vi "helper-log-visa.vi"(11 "VISA REPORT":T2) -> (0 "error out":errorcluster, 3 "array type (2D Dbl)":string[][](array[string]))   [LabVIEW 2024]
uses:
  controls/enum.io.type.ctl
  controls/enum.report-filter.ctl
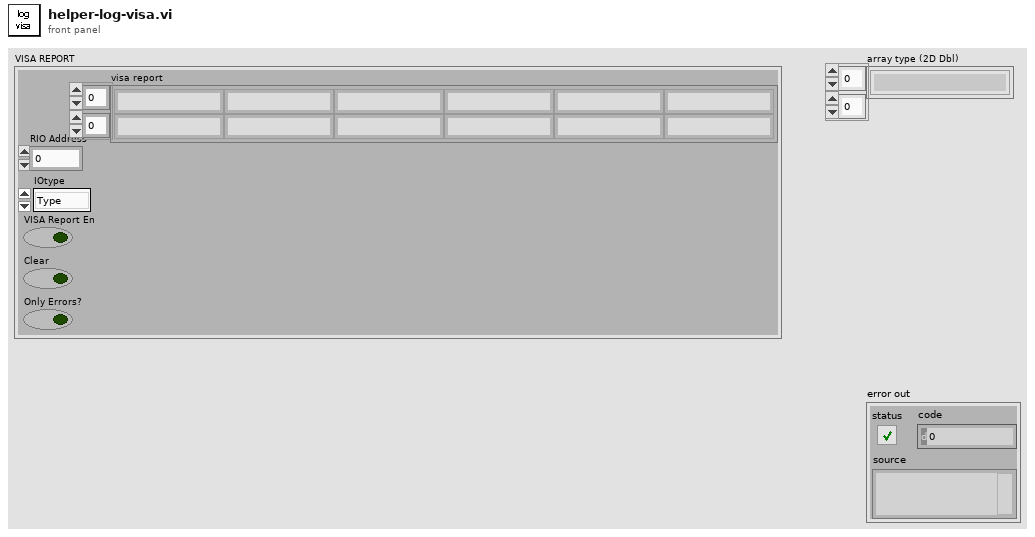
[diagram p1: front panel]
types:
  T1 = typedef "enum.io.type.ctl" = enum16{"Type", "DI", "DO", "AI", "AO", "VL", "BUF"}
  T2 = cluster{"visa report":string[][], "RIO Address":i32, "IOtype":T1, "VISA Report En":bool, "Clear":bool, "Only Errors?":bool}
  T3 = typedef "enum.report-filter.ctl" = enum16{"Read ALL", "Read Errors", "Collect", "ClearAll"}
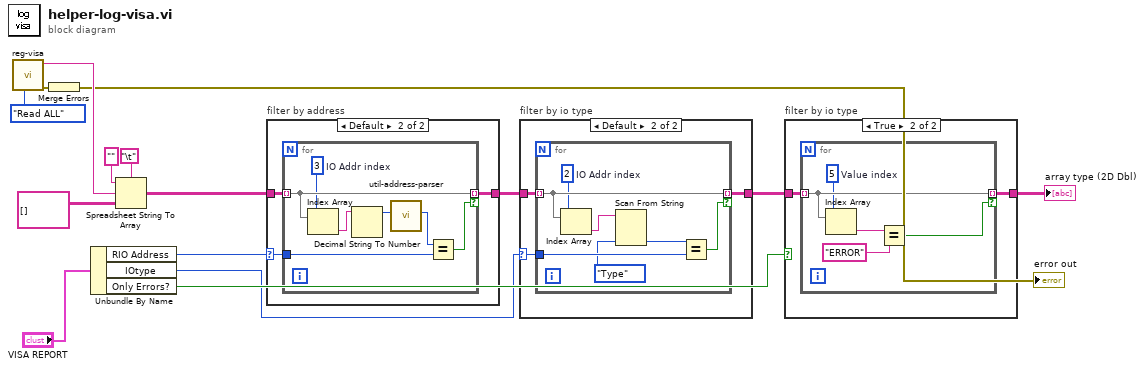
[diagram p0: block diagram]
diagram:
  n1 = call "reg-visa.vi"("Operation(Read)"=enum.report-filter."Read ALL") -> ("error out"=w3:errorcluster, "Collected Reports"=w6:string)  [unwired: 9 in]
  n2 = Merge Errors(w3) -> (→"error out":errorcluster)
  n3 = Unbundle By Name("VISA REPORT") -> ("RIO Address"=w9:i32, "IOtype"=w10:T1, "Only Errors?"=w13:bool)
  n4 = Spreadsheet String To Array(delimiter (Tab)="\t", format string="", spreadsheet string=w6, array type (2D Dbl)=string[][] []) -> (array=w5:string[][])
  n5 = case "filter by address" shown="Default" w9 {
    selector: w9 -> [_ w18]
    tunnel: w5 -> [w16 w19]
    tunnel: [w16 w17] -> w11
    frame ..0 {
    }
    frame Default {
      n6 = for {
        tunnel: w19 -> [w22] mode=indexing
        tunnel: w18 -> [w23]
        tunnel: [w22] -> w17 mode=indexing if=w21
        w20 = 3  # IO Addr index
        n7 = Index Array(array=w22, index=w20) -> (element=w26:string)
        n8 = Decimal String To Number(string=w26) -> (number=w25:i32)  [unwired: 2 in, 1 out]
        n9 = call "util-address-parser.vi"("ADDR 2"=w25) -> ("Address"=w24:u8)  [unwired: 9 in, 1 out]
        n10 = Equal?(x=w24, y=w23) -> (x = y?=w21:bool)
      }
    }
  }
  n11 = case "filter by io type" shown="Default" w10 {
    selector: w10 -> [_ w29]
    tunnel: w11 -> [w27 w30]
    tunnel: [w27 w28] -> w14
    frame "Type" {
    }
    frame Default {
      n12 = for {
        tunnel: w30 -> [w37] mode=indexing
        tunnel: w29 -> [w33]
        tunnel: [w37] -> w28 mode=indexing if=w36
        w35 = 2  # IO Addr index
        n13 = Index Array(array=w37, index=w35) -> (element=w34:string)
        n14 = Scan From String(input string=w34, default 1=enum.io.type."Type" ("IOtype")) -> (output 1=w32:T1)  [unwired: 3 in, 3 out]
        n15 = Equal?(x=w32, y=w33) -> (x = y?=w36:bool)
      }
    }
  }
  n16 = case "filter by io type" shown="True" w13 {
    tunnel: w14 -> [w38 w40]
    tunnel: [w38 w39] -> w15
    frame False {
    }
    frame True {
      n17 = for {
        tunnel: w40 -> [w45] mode=indexing
        tunnel: [w45] -> w39 mode=indexing if=w44
        w43 = 5  # Value index
        n18 = Index Array(array=w45, index=w43) -> (element=w42:string)
        n19 = Equal?(x=w42, y="ERROR") -> (x = y?=w44:bool)
      }
    }
  }
  "array type (2D Dbl)" <- w15
